vi "Keithley Fres.vi"(2 "Delay":dbl, 3 "Average Measurements":dbl, 4 "VISA resource name":refnum<visa-resource-name>) -> (1 "Resistance":dbl)   [LabVIEW 2014]
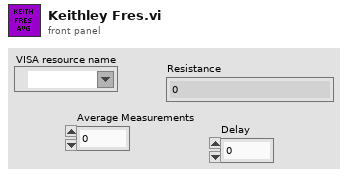
[diagram p1: front panel]
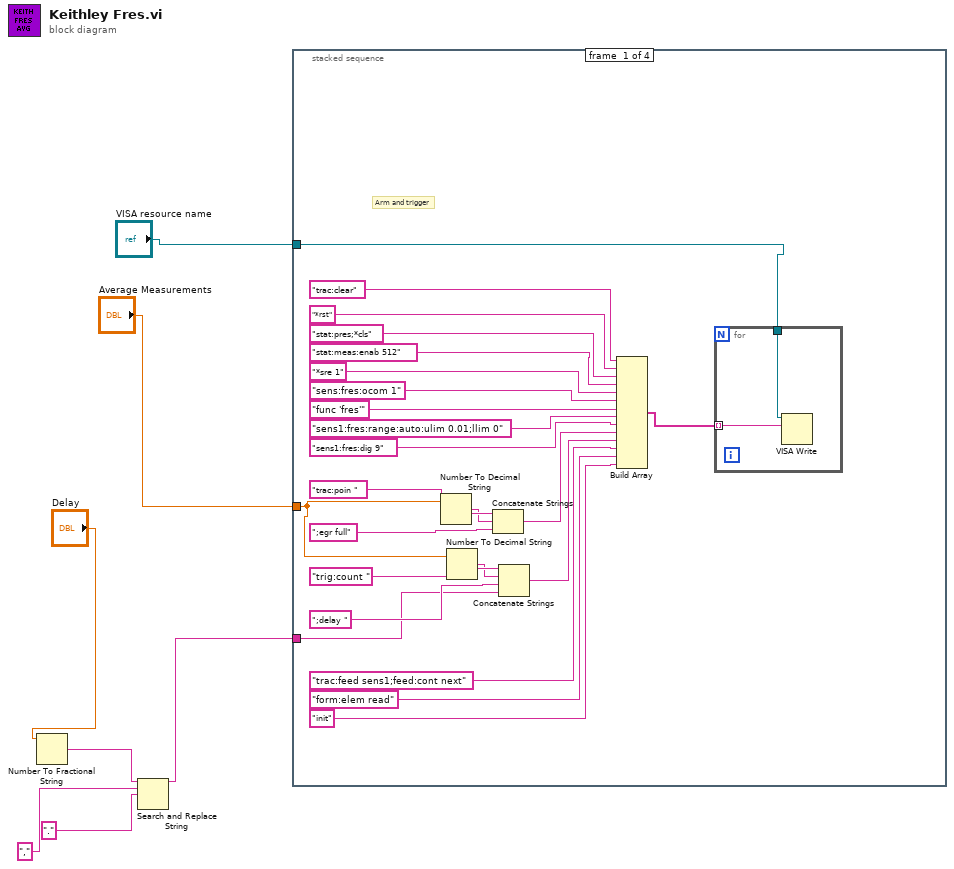
[diagram p0: block diagram]
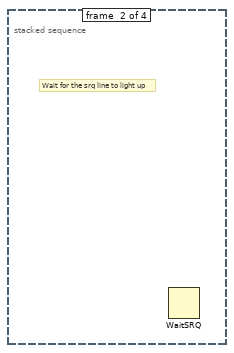
[diagram p2: hidden frame]
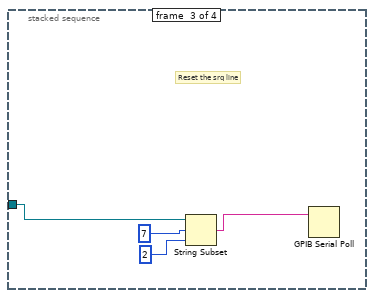
[diagram p3: hidden frame]
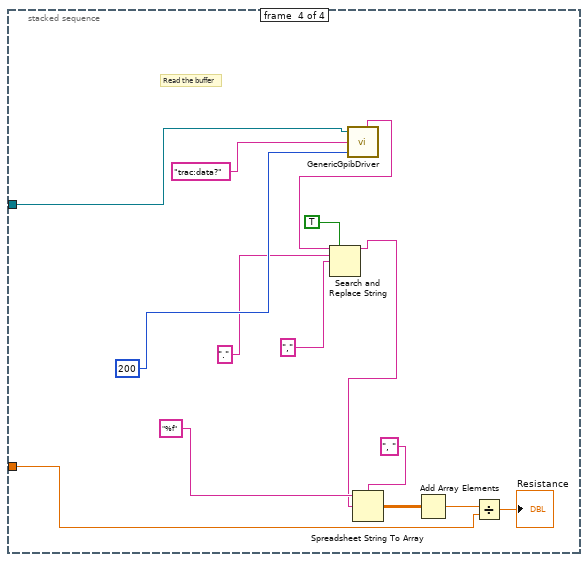
[diagram p4: hidden frame]
diagram:
  n1 = Number To Fractional String(number="Delay") -> (F-format string=w5:string)  [unwired: 3 in]
  n2 = Search and Replace String(input string=w5, search string=",", replace string=".") -> (result string=w1:string)  [unwired: 5 in, 3 out]
  n3 = stacked-sequence {
    tunnel: "VISA resource name" -> [w18 _ w35 w49]
    tunnel: "Average Measurements" -> [w10 _ _ w38]
    tunnel: w1 -> [w8 _ _ _]
    frame #0 {
      # "Arm and trigger"
      n4 = Number To Decimal String(number=w10) -> (decimal integer string=w16:string)  [unwired: 1 in]
      n5 = Number To Decimal String(number=w10) -> (decimal integer string=w12:string)  [unwired: 1 in]
      n6 = Concatenate Strings("trac:poin ", w16, ";egr full") -> (w14:string)
      n7 = Concatenate Strings("trig:count ", w12, ";delay ", w8) -> (w9:string)
      n8 = Build Array("trac:clear", "*rst", "stat:pres;*cls", "stat:meas:enab 512", "*sre 1", "sens:fres:ocom 1", "func 'fres'", "sens1:fres:range:auto:ulim 0.01;llim 0", "sens1:fres:dig 9", w14, w9, "trac:feed sens1;feed:cont next", "form:elem read", "init") -> (w30:string[])
      n9 = for {
        tunnel: w30 -> [w33] mode=indexing
        tunnel: w18 -> [w32]
        n10 = VISA Write(VISA resource name=w32, write buffer=w33) -> ()  [unwired: 1 in, 3 out]
      }
    }
    frame #1 {
      # "Wait for the srq line to light up"
      n11 = WaitSRQ() -> ()  [unwired: 2 in, 3 out]
    }
    frame #2 {
      # "Reset the srq line"
      n12 = String Subset(string=w35, offset (0)=7, length (rest)=2) -> (substring=w34:string)
      n13 = GPIB Serial Poll(0:w34) -> ()  [unwired: 1 in, 3 out]
    }
    frame #3 {
      # "Read the buffer"
      n14 = call "GenericGpibDriver.vi"("Wait (ms)"=200, "Command"="trac:data?", "VISA resource name"=w49) -> ("Return Value"=w48:string)  [unwired: 1 in, 4 out]
      n15 = Search and Replace String(replace all?=TRUE ("replace all? (F)"), input string=w48, search string=".", replace string=",") -> (result string=w43:string)  [unwired: 4 in, 3 out]
      n16 = Spreadsheet String To Array(delimiter (Tab)=", ", format string="%f", spreadsheet string=w43) -> (array=w41:dbl[][])  [unwired: 1 in]
      n17 = Add Array Elements(numeric array=w41) -> (sum=w40:dbl)
      n18 = Divide(x=w40, y=w38) -> (x/y=→"Resistance":dbl)
    }
  }
